vi "Device and User PGSQL Paths.vi"(7 "instrument":T1=enum."PPMS 1") -> (2 "User Path":string, 3 "Device Path":string)   [LabVIEW 2016, in "Control Experiment SM.lvclass"]
uses:
  Control Experiment SM.lvclass
  Typedefs/Instrument--enum.ctl
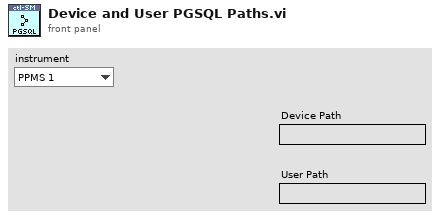
[diagram p1: front panel]
types:
  T1 = typedef "Control Experiment SM.lvclass/Instrument--enum.ctl" = enum16{"----- AFM/EBL -----", "AGILENT", "CYPHER", "Gemini2", "JEOL", "MFP3D", "----- Cryostat -----", "CF900", "DR200", "MNK", "PPMS 1", "PPMS 2", "PPMS 3", "----- Optics -----", "THz 1", "THz 2"}
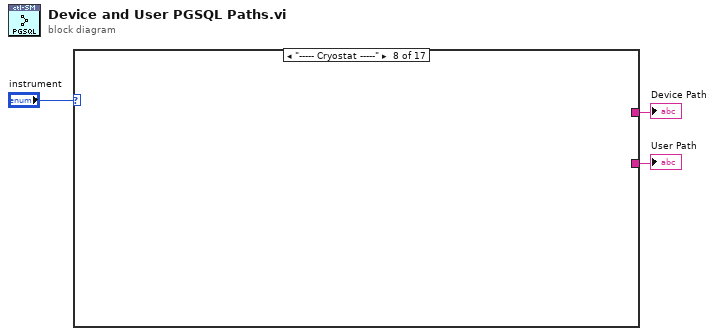
[diagram p0: block diagram]
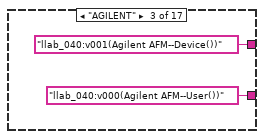
[diagram p4: hidden frame]
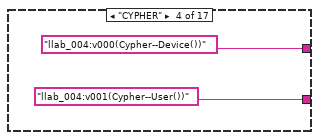
[diagram p5: hidden frame]
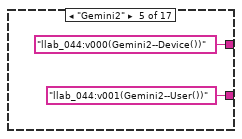
[diagram p6: hidden frame]
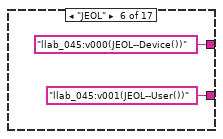
[diagram p7: hidden frame]
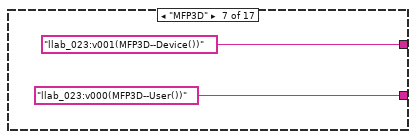
[diagram p8: hidden frame]
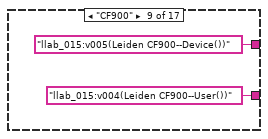
[diagram p9: hidden frame]
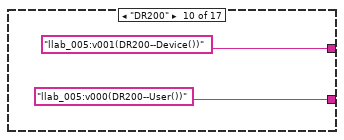
[diagram p10: hidden frame]
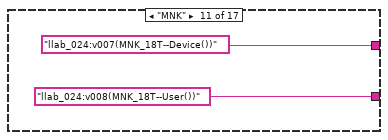
[diagram p11: hidden frame]
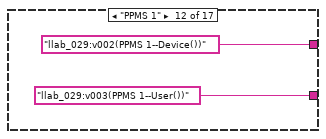
[diagram p12: hidden frame]
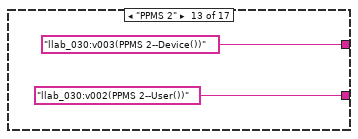
[diagram p13: hidden frame]
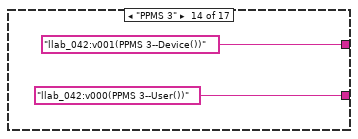
[diagram p14: hidden frame]
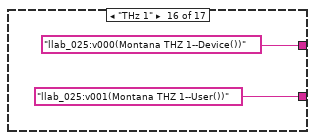
[diagram p16: hidden frame]
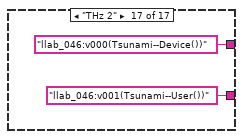
[diagram p17: hidden frame]
diagram:
  n1 = case shown="\"----- Cryostat -----\"" "instrument" {
    tunnel: [_ _ "llab_040:v001(Agilent AFM--Device())" ("Device Path") "llab_004:v000(Cypher--Device())" ("Device Path") "llab_044:v000(Gemini2--Device())" ("Device Path") "llab_045:v000(JEOL--Device())" ("Device Path") "llab_023:v001(MFP3D--Device())" ("Device Path") _ "llab_015:v005(Leiden CF900--Device())" ("Device Path") "llab_005:v001(DR200--Device())" ("Device Path") "llab_024:v007(MNK_18T--Device())" ("Device Path") "llab_029:v002(PPMS 1--Device())" ("Device Path") "llab_030:v003(PPMS 2--Device())" ("Device Path") "llab_042:v001(PPMS 3--Device())" ("Device Path") _ "llab_025:v000(Montana THZ 1--Device())" ("Device Path") "llab_046:v000(Tsunami--Device())" ("Device Path")] -> w2
    tunnel: [_ _ "llab_040:v000(Agilent AFM--User())" ("Device Path") "llab_004:v001(Cypher--User())" ("Device Path") "llab_044:v001(Gemini2--User())" ("Device Path") "llab_045:v001(JEOL--User())" ("Device Path") "llab_023:v000(MFP3D--User())" ("Device Path") _ "llab_015:v004(Leiden CF900--User())" ("Device Path") "llab_005:v000(DR200--User())" ("Device Path") "llab_024:v008(MNK_18T--User())" ("Device Path") "llab_029:v003(PPMS 1--User())" ("Device Path") "llab_030:v002(PPMS 2--User())" ("Device Path") "llab_042:v000(PPMS 3--User())" ("Device Path") _ "llab_025:v001(Montana THZ 1--User())" ("Device Path") "llab_046:v001(Tsunami--User())" ("Device Path")] -> w1
    frame Default {
    }
    frame "----- AFM/EBL -----" {
    }
    frame "AGILENT" {
    }
    frame "CYPHER" {
    }
    frame "Gemini2" {
    }
    frame "JEOL" {
    }
    frame "MFP3D" {
    }
    frame "----- Cryostat -----" {
    }
    frame "CF900" {
    }
    frame "DR200" {
    }
    frame "MNK" {
    }
    frame "PPMS 1" {
    }
    frame "PPMS 2" {
    }
    frame "PPMS 3" {
    }
    frame "----- Optics -----" {
    }
    frame "THz 1" {
    }
    frame "THz 2" {
    }
  }
  "Device Path" <- w2
  "User Path" <- w1
